vi "Transmit.vi"(8 "error in (no error)":errorcluster, 9 "timeout in ms (-1)":i32=-1, 10 "Packet Data":u8[](array[numeric]), 11 "Local Queues in":T1) -> (0 "error out":errorcluster, 1 "Timeout?":bool, 2 "Packet Data Sent":u8[](array[numeric]), 3 "Local Queues out":T1)   [LabVIEW 2020, in "Communication VIs.lvlib" / "Local.lvlib"]
uses:
  Local.lvlib
  Local Queues.ctl
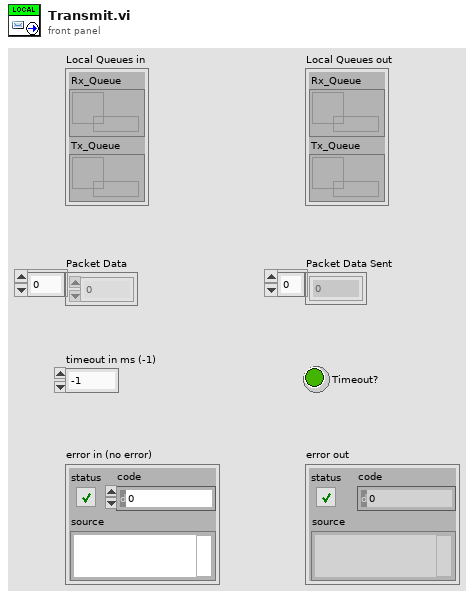
[diagram p1: front panel]
types:
  T1 = typedef "Communication VIs.lvlib/Local.lvlib/Local Queues.ctl" = cluster{"Rx_Queue":refnum<queue>, "Tx_Queue":refnum<queue>}
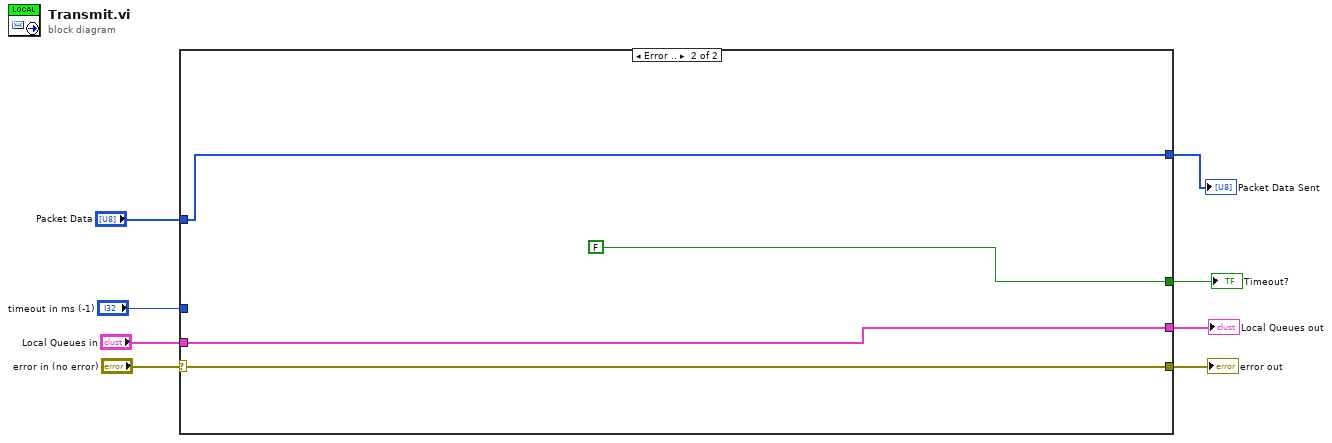
[diagram p0: block diagram]
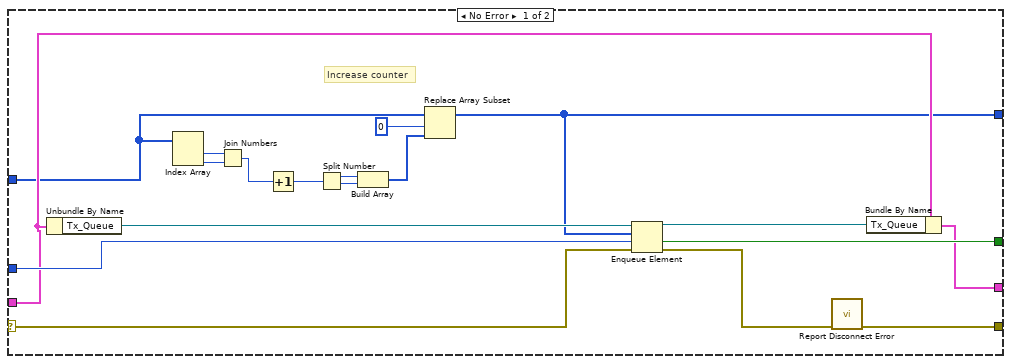
[diagram p2: hidden frame]
diagram:
  n1 = case shown="Error .." "error in (no error)" {
    selector: "error in (no error)" -> [w25 w30]
    tunnel: "timeout in ms (-1)" -> [w26 _]
    tunnel: [w22 w30] -> w8
    tunnel: [w27 FALSE ("timed out?")] -> w7
    tunnel: "Local Queues in" -> [w21 w29]
    tunnel: [w19 w29] -> w3
    tunnel: "Packet Data" -> [w10 w28]
    tunnel: [w9 w28] -> w1
    frame No Error {
      # "Increase counter"
      n2 = Unbundle By Name(w21) -> ("Tx_Queue"=w24:refnum<queue>)
      n3 = Index Array(array=w10) -> (element #1=w13:u8, element #2=w12:u8)  [unwired: 2 in]
      n4 = Join Numbers(hi=w13, lo=w12) -> ((hi.lo)=w11:u16)
      n5 = Increment(x=w11) -> (x+1=w14:u16)
      n6 = Split Number(x=w14) -> (hi(x)=w18:u8, lo(x)=w17:u8)
      n7 = Build Array(w18, w17) -> (w16:u8[])
      n8 = Replace Array Subset "Replace Array Subset"(array=w10, new element=w16, index=0) -> (w9:u8[])
      n9 = Enqueue Element(queue=w24, element=w9, timeout in ms (-1)=w26, error in (no error)=w25) -> (queue out=w20:refnum<queue>, timed out?=w27:bool, error out=w23:errorcluster)
      n10 = call "Report Disconnect Error.vi"("error in (no error)"=w23) -> ("error out"=w22:errorcluster)  [unwired: 10 in]
      n11 = Bundle By Name(cluster=w21, "Tx_Queue"=w20) -> (w19:T1)
    }
    frame Error {
    }
  }
  "error out" <- w8
  "Timeout?" <- w7
  "Local Queues out" <- w3
  "Packet Data Sent" <- w1
